vi "UHR-Fleezers Control (host) - 10.4.vi"() -> ()   [LabVIEW 2011] (continued)
  out "Progress":u16(slide) scale=0.0..100.0
  out "Manipulating Trap":bool
  out "Buffer Status":dbl(slide) scale=0.0..1.0
  out "Overflow (data lost)":bool
  in  "Reset":bool
  out "Data Rate (Hz)":dbl=66666.66666666667 caption="Trap Data Rate (Hz)" format="%#_3p"
  out "Data Period (s)":dbl=1.4999999999999999e-05 caption="Trap Data Period (s)" format="%#_6p"
  out "Save Data Rate (Hz)":dbl=133.33333333333334 caption="Rate (Hz)" format="%#_6p"
  out "Save Data Period (s)":dbl=0.0075 caption="Period (s)" format="%#_6p"
  in  "T1 alpha_x (nm/V)":dbl=624.3667930897869 step=10.0 format="%#_3g"
  in  "T2 alpha_x (nm/V)":dbl=812.659816494575 step=10.0 format="%#_3g"
  in  "T2 kappa_x (pN/nm)":dbl=0.20437519788264086 min=0.0 step=0.001 format="%#_2g"
  in  "T2 offset_x (mV)":dbl=53.075312649641084 format="%#_2g"
  in  "BD 1 Frequency 1 (MHz)":dbl=70.0 caption="T1 X (MHz)" min=60.0 max=90.0 step=1.0 format="%#_6p"
  in  "BD 1 Frequency 2 (MHz)":dbl=85.0 caption="T2 X (MHz)" min=60.0 max=90.0 step=1.0 format="%#_6p"
  in  "Green Laser ON/Interlacing":bool
  in  "Round T2 X":bool caption="Round"
  in  "AO1":dbl(slide)=7.146906643879515 caption="Confocal Y (V)" min=0.0 max=10.0 step=0.01 scale=0.0..10.0 scale format="%_1f"
  in  "AO2":dbl(slide)=1.424915616321299 caption="Confocal X (V)" min=0.0 max=10.0 step=0.01 scale=0.0..10.0 scale format="%_1f"
  in  "Trap Raster Scan":bool
  out "Raster Scanning...":bool
  in  "Trap Delta (MHz)":dbl=15.0
  in  "Setpoints (V)":cluster{"Set 1":dbl, "Set 2":dbl}={"Set 1"=9.0, "Set 2"=9.0}
  in  "Green FB Setpoint (mV)":dbl=200.0
  in  "Fish for Tether":bool
  in  "Position Label 5":string="upper flow spot (UvrD)" caption="5"
  in  "Move to Position":bool
  in  "Position":dbl=1.0 min=1.0 max=10.0 step=1.0
  in  "Set Position":bool
  in  "Saved Stage Positions":dbl[][](array[numeric])=[[1.0, 0.0, 0.0, 0.0], [2.0, -0.38428, -2.10668, -0.02109], [3.0, 1.5, -0.5, 0.0], [4.0, -0.59033, -2.08842, -0.03013], [5.0, 1.5, -2.25, 0.0], [6.0, 0.0, 0.0, 0.0], [7.0, 0.0, 0.0, 0.0], [8.0, 0.0, 0.0, 0.0], [9.0, 0.0, 0.0, 0.0], [10.0, 0.0, 0.0, 0.0]]
  in  "Move to Position 5":bool
  in  "z nudge increment (um)":dbl=0.5
  in  "+z":bool
  in  "Position 1 Label":string="Lower capillary (DNA beads)" caption="1"
  in  "Set Position 1":bool
  in  "Set Position 2":bool
  in  "Set Position 3":bool
  in  "Set Position 4":bool
  in  "Move to Position 3":bool
  in  "Move to Position 4":bool
  in  "Move to Position 2":bool
  in  "Move to Position 1":bool
  in  "Position 2 Label":string="Upper capillary (ADig beads)" caption="2"
  in  "Position 3 Label":string="lower flow spot (ATP)" caption="3"
  in  "Position 4 Label":string="Dump beads" caption="4"
  in  "-z":bool
  in  "Set Position 5":bool
  out "Stage Control Serial Error":errorcluster={"status"=FALSE, "code"=1073676293, "source"="VISA Read in Set Stage Position.vi->UHR-Fleezers Control (host) - 10.4.vi"}
  in  "Clear Volume":bool caption="Clear Infused Volume"
  in  "Flow rate (uL/h)":dbl=100.0
  in  "Flush rate (uL/m)":dbl=100.0
  out "Pump 3 cont disp":string="Left: ADig beads"
  out "Pump 1 cont disp":string="Right: DNA beads "
  in  "Ch 1 Inject Rate (ul/h)":dbl=1600.0
  in  "Pump write delay (ms)":dbl=300.0
  in  "All Pump Parameters":T5={"Pump 1"={"Diameter (mm)"=4.61, "Units"=4.0, "Volume"=100.0, "Rate"=1600.0}, "Pump 2"={"Diameter (mm)"=4.61, "Units"=3.0, "Volume"=0.0, "Rate"=0.0}, "Pump 3"={"Diameter (mm)"=4.61, "Units"=4.0, "Volume"=100.0, "Rate"=800.0}}
  in  "Ch 1 Inject Volume (uL)":dbl=100.0
  in  "Pump pause delay (ms)":u32
  in  "Ch 3 Inject Volume (uL)":dbl=100.0
  in  "Ch 3 Inject Rate (ul/h)":dbl=800.0
  in  "Flush Center Ch Volume (uL)":dbl=15.0
  in  "Flush Center Ch Rate (ul/m)":dbl=100.0
  in  "Inject Pump 2":bool caption="Inject Pump 2\n(Flush Center)"
  in  "Total Volume\nFlushed (uL)":dbl
  in  "Flush Sample":bool
  in  "Volume (uL)":dbl=100.0
  in  "Tab Control 2":T6(tab)=enum."Feedback on Trap Position"
  out "Total Counts (ticks)":u32=600
  in  "Trap ON/OFF X or Y Amp?":bool=TRUE
  in  "Oscillate Set 1":bool
  in  "Trap 1 ON":bool=TRUE
  in  "Number Interlace Sets":u8=3 min=1 max=3
  in  "DIO count 3 (ticks)":u32=200
  in  "DIO count 2 (ticks)":u32=200
  in  "DIO count 1 (ticks)":u32=200
  in  "BD 2 Amplitude 3 (%)":dbl min=0.0 max=50.0 step=1.0
  in  "BD 2 Amplitude 2 (%)":dbl min=0.0 max=50.0 step=1.0
  in  "BD 2 Amplitude 1 (%)":dbl min=0.0 max=50.0 step=1.0
  in  "BD 1 Amplitude 3 (%)":dbl min=0.0 max=50.0 step=1.0
  in  "BD 1 Amplitude 2 (%)":dbl=35.0 min=0.0 max=50.0 step=1.0
  in  "BD 1 Amplitude 1 (%)":dbl=10.0 min=0.0 max=50.0 step=1.0
  in  "BD 2 Frequency 3 (MHz)":dbl=26.0 min=0.0 max=40.0 step=1.0 format="%#_6p"
  in  "BD 1 Frequency 3 (MHz)":dbl=70.0 min=60.0 max=90.0 step=1.0 format="%#_6p"
  in  "BD 2 Frequency 2 (MHz)":dbl=26.0 min=0.0 max=40.0 step=1.0 format="%#_6p"
  in  "BD 2 Frequency 1 (MHz)":dbl=26.0 min=0.0 max=40.0 step=1.0 format="%#_6p"
  in  "Not-Interlacing Set":enum32{"Set 1", "Set 2", "Set 3"}(radio)
  in  "Interlace":bool=TRUE
  in  "Trap 2 ON":bool
  in  "Trap 3 ON":bool
  in  "Scan axis 2":bool=TRUE
  in  "Osc. freq. (Hz)":dbl=0.25
  in  "Osc. amp. (MHz)":dbl=2.0
  out "Coords":T7
  in  "Manipulation Scaling":cluster{"Horizontal":dbl, "Vertical":dbl}={"Horizontal"=0.075, "Vertical"=0.01}
  in  "Freq or Amp switch first":bool=TRUE
  in  "Swap F1 and F2":bool
  in  "Freq switch delay":u16
  in  "Amp switch delay":u16=5
  in  "MCL Step Increment (V_int)":dbl=3.0
  out "Time to Finish All (min)":dbl=0.13986 format="%#_2p"
  in  "Scan Speed (nm/s)":dbl=100.0
  in  "Scan Range (nm)":dbl=420.0
  in  "Step Size (nm)":dbl=1.0
  in  "MCL/AOM Scale Tweak":dbl=1.0
  in  "MCL Step Position Ratio":dbl=0.5
  in  "Move MCL Also?":bool=TRUE
  out "Final sep (nm)":dbl=1440.000000000001
  out "Initial sep (nm)":dbl=1020.0
  out "Save index":dbl=12.0
  out "Final delta (MHz)":dbl=18.41463414634147
  out "Initial delta (MHz)":dbl=15.0
  out "Final freq. (MHz)":dbl=66.58536585365853
  out "Initial freq. (MHz)":dbl=70.0
  in  "Saved AOD Raster Scan Parameter Sets":T8(array[cluster])=[{"Scan Range AOD (nm) 2"=500.0, "Step Size AOD (nm) 2"=1.0, "Scan Speed AOD (nm/s) 2"=100.0, "Number of scans (AOD) 2"=1, "Label"="offset curve"}, {"Scan Range AOD (nm) 2"=420.0, "Step Size AOD (nm) 2"=1.0, "Scan Speed AOD (nm/s) 2"=100.0, "Number of scans (AOD) 2"=1, "Label"="hp raster check"}, {"Scan Range AOD (nm) 2"=6.8, "Step Size AOD (nm) 2"=0.34, "Scan Speed AOD (nm/s) 2"=0.34, "Number of scans (AOD) 2"=1, "Label"="3.4 kbp - 1 bp steps"}, {"Scan Range AOD (nm) 2"=215.0, "Step Size AOD (nm) 2"=1.0, "Scan Speed AOD (nm/s) 2"=100.0, "Number of scans (AOD) 2"=3, "Label"="dt14 1 14 MHz start"}, {"Scan Range AOD (nm) 2"=450.0, "Step Size AOD (nm) 2"=1.0, "Scan Speed AOD (nm/s) 2"=100.0, "Number of scans (AOD) 2"=1, "Label"="dt14 2 small beads"}]
  in  "Load parameters":bool
  out "Scan Range (MHz)":dbl=-3.4146341463414633
  in  "Restart DMA? (AOD)":bool=TRUE caption="Restart DMA?"
  out "Incr. int (AOD)":i64=-7759651845
  out "Time/Scan (s) (AOD)":dbl=4.1958 format="%#_2p"
  out "Data points/scans":dbl=559440.0
  out "Data points/scan (f/b)":dbl=559440.0
  in  "Save scans":bool=TRUE
  out "AOD Scan I":u64=2 caption="Scan I"
  in  "Continuous AOD Scanning":bool caption="Continuous Scanning"
  in  "Abort AOD Scan":bool caption="Abort Scan"
  in  "Scan BD":bool=TRUE
  out "Cycles/step (AOD)":u64=666 format="%.3p"
  in  "Number of F/B Scans (AOD)":u16=1 min=1
  out "Scan steps (AOD)":u64=420
  out "Scan Increment (MHz)":dbl=-0.008149484836137144
  out "AOD Scanning":bool caption="Scanning"
  in  "Start AOD Scan":bool caption="Start Scan"
  out "N sets should be saved":dbl=27.972
  out "Progress 2":u16(slide) caption="Progress" scale=0.0..100.0
  in  "Abort save 2":bool caption="Abort save"
  in  "Trap 1 Bead Size (nm)":dbl=860.0
  in  "Trap 2 Bead Size (nm)":dbl=790.0
  out "MCL Count":dbl=782931.6080202643
  in  "All FB On/Off":bool=TRUE
  in  "AI2 to Setpoint":cluster{"Set 1":bool, "Set 2":bool}
  out "AI2 (V)":cluster{"Set 1":dbl, "Set 2":dbl}={"Set 1"=9.049958800012208, "Set 2"=0.022888882106997896}
  in  "Reset Feedback":cluster{"Set 1":bool, "Set 2":bool}
  in  "PID Gains":T9={"Set 1"={"proportional gain (Kc)"=0, "integral gain (Kc*Ts/Ti)"=5, "derivative gain (Kc*Td/Ts)"=0}, "Set 2"={"proportional gain (Kc)"=0, "integral gain (Kc*Ts/Ti)"=5, "derivative gain (Kc*Td/Ts)"=0}}
  in  "Feedback On/Off":cluster{"Set 1":bool, "Set 2":bool}={"Set 1"=TRUE, "Set 2"=TRUE}
  in  "Rem fb disp offset":bool caption="Rem. Offset"
  in  "Remove Unwinding Offset":bool
  in  "FB Trap Pos Offset":dbl=-32.20986371566535 caption="Offset (nm)" format="%.1f"
  in  "Negate Y Axis":bool=TRUE
  in  "Set Reading to\nSetpoint":bool
  out "Trap X (AI1)":T10={"Trap 1"=0.05029296875, "Trap 2"=-0.09722900390625}
  in  "Trap Pos FB SP":fxp<+/-,16,1>=-0.008514404296875 caption="Setpoint"
  in  "Trap Pos. FB ON":bool
  in  "Reset Trap Pos. FB":bool
  out "Trap Positions":waveform(dbl)[](graph)=[{"t0"=timestamp(5315.100000001762 s since 1904-01-01), "dt"=0.15, "Y"=[-32.20986371563738, -32.20986371563738], "attributes"=variant("NI_ChannelName"=variant(string "Trap 1 Pos."))}, {"t0"=timestamp(5315.100000001762 s since 1904-01-01), "dt"=0.15, "Y"=[-5.5933924159035087e-11, -5.5933924159035087e-11], "attributes"=variant("NI_ChannelName"=variant(string "Trap 2 Pos."))}]
  in  "Tab Control 8":enum32{"Main Setting", "Details"}(tab)
  in  "Trap Pos FB Int Count":u16=100
  in  "Trap Pos. FB Gains":T11={"proportional gain (Kc)"=10.0, "integral gain (Kc*Ts/Ti)"=10.0, "derivative gain (Kc*Td/Ts)"=0.0} {"proportional gain (Kc)" format="%.11g"; "integral gain (Kc*Ts/Ti)" format="%.11g"; "derivative gain (Kc*Td/Ts)" format="%.11g"}
  in  "Trap Pos. FB Offset Factor":i64
  in  "Trap Pos FB Negate Action":bool
  in  "Trap Pos. FB Mult Factor":i64=33554432
  in  "Trap Pos. AI1 X Pre-scale":u16
  in  "Trap Pos. FB Range":T12={"output high"=0.999969482421875, "output low"=-1.0}
  out "Trap Pos FB Int Signal":fxp<+/-,24,9>=-1.02886962890625 format="%.18g"
  out "Trap Pos FB Int-Norm Signal":fxp<+/-,16,1>=-0.010284423828125 format="%.16g"
  in  "Set SP Using...":bool
  in  "Trap Pos FB Monitor\nT1 or T2":bool
  out "Trap X AI1 (DMA)":T13={"Set 1"=0.05328369140625, "Set 2"=-0.139556884765625}
  in  "N El. to Ave.":dbl=10000.0
  out "Trap Pos FB Action":i64=23570
  out "Action (%)":dbl(knob)=71.93212683492538 scale=-100.0..100.0
  in  "Trap Pos. FB Out Scale 2^n":u8=25 caption="Action Scale Factor"
  out "Mean T1 Position (nm)":dbl=-32.20986371563738 caption="Mean T1 (nm)" format="%0.2f"
  out "Trap 1 Position RMS (A)":dbl caption="RMS (Ang)"
  in  "Remove Action Offset":bool
  in  "factor":dbl=0.8
  in  "Trap Pos. Disp. Downsample":dbl=10000.0 caption="Trap Downsample"
  in  "Tab Control 3":enum32{"Timing", "MCL Scan", "Analog Out"}(tab)
  out "APD 2 Gate Late Counter":u32
  out "APD 2 Gate Relative Phase":i16
  in  "Phase Adj. (APD 2 Gate)":i16=20
  in  "Initial Phase Adjustment (APD 2 Gate)":i16=55
  out "APD 1 Gate Late Counter":u32
  in  "- phase (APD 1 Gate)":bool
  in  "+ phase (APD 1 Gate)":bool
  out "APD 1 Gate Relative Phase":i16
  in  "Phase Adj. (APD 1 Gate)":i16=20
  in  "Initial Phase Adjustment (APD 1 Gate)":i16=60
  in  "Save APD Data\nwith Trap Data":bool=TRUE
  out "APD FIFO Elements Remaining":u32
  in  "- phase (APD Acq)":bool
  in  "+ phase (APD Acq)":bool
  out "APD Acq Late Counter":u32
  out "APD Acq Relative Phase":i16
  in  "Phase Adj. (APD Acq)":i16=20
  in  "Initial Phase Adjustment (APD Acq)":i16
  in  "Invert APD Gate":bool caption="Invert Gate"
  in  "APD Gate OFF Count":u32=450 caption="Gate OFF Count"
  in  "APD Gate ON Count":u32=150 caption="Gate ON Count"
  in  "APD Gate":enum32{"ON", "OFF", "Interlace"}(radio)=enum."Interlace"
  in  "APD Integration Time (s)":dbl=0.01 caption="Integration Time (s)"
  out "APD Acq Rate (Hz)":dbl=100.0 caption="Rate (Hz)"
  out "APD Samples/FIFO Acq.":dbl=30.0
  out "APD Elements/DMA read":u32=60
  out "APD Int. Count":u32=400000 format="%.0p"
  in  "+ phase (APD 2 Gate)":bool
  in  "- phase (APD 2 Gate)":bool
  in  "Tab Control 5":enum32{"PSD X", "PSD Y", "Other Data Channel"}(tab)
  out "Data map":dbl[][](graph)=[[0.001974800723796629, -0.0013307077949780925, 3.5478396375182556e-05, -0.0008656630334600533, 0.003722726291225046, 0.0009559614811579494, 0.0004067776954783719, -0.0005330988948040376, -0.001176093052158523, 0.0004508069091133665, -0.0009073488729753098, -0.0007052486419013018, 0.00020789655803253064, 0.0001241869508331131, 0.0037172511150124366, -0.0002939967002449287, -0.00015207858051379504, -9.320397918003548e-05, -4.818930038232472e-05, 0.0003043649821186849], [-0.001031665574705379, -0.0005831254477400646, 0.0012531205354473264, 0.0006867260941382034, 0.00039068341874680536, -0.0008665544113564399, 1.1155677774738132e-05, -0.0004058382977629158, -0.0007996984738111764, 0.0006720220745334646, -5.2295719559871024e-05, 0.0020160741300127927, 0.0011086934717958095, 0.00022784846412103992, 0.0014286413450522995, -0.000625478515904662, -0.00032260854393552883, 0.0014821578105266167, -0.0006624520387635512, -0.0008196499516340234], [0.0008707462370312414, 0.0008734847802455585, -0.0009375270569827855, -0.0005301325848379493, 0.0008581834048839196, -0.00038982434612128277, 0.003239773338572745, -0.00020397792231700303, 0.0007502371285024098, 0.0002674083017176036, 0.0006760027114216932, -0.0005268526629850034, -0.0008874403582654871, 0.0021340380967751838, 0.00038914081701392413, -0.000607773836931023, 0.00040958612136905335, -8.912906425596873e-05, -0.000978322721709446, -0.0004259412094274336], [0.0010167653949750284, -0.001227712955400397, -0.0005828111751727386, -0.00034681313733748873, 0.0011154140304214628, 0.0009698055107082625, 0.0003047086624579304, -0.000896404784165975, 0.0010714187743685885, 0.0003983374192823886, -4.912248607555678e-05, -1.2318516008092849e-05, 9.095897165929441e-05, 0.0015280892564470835, 0.0015086948659084063, -0.0002666063281217702, -0.00023529227277871242, -0.00036125092589777287, -0.0014159788458990696, -2.710729292442805e-05], [-8.167246872768262e-05, 0.0009598305190754163, 0.0003747131180220494, 0.0012690684222979877, -0.00034832954634158697, 5.649447215263457e-05, 0.0004890411957727576, -0.0007578336539554914, -0.00040934283442915705, 0.0007452279948579076, 0.00015620465662804465, 0.0018487220354370564, 0.0014080398272018054, -0.00041784730224639767, -0.0003903906172355312, -0.0003199149811349592, 0.00035618530065829087, -0.0006799972758753446, -0.0003889301678648796, -0.0005956701562327435], [0.0018039939622592623, 0.0005245361826948688, -0.0005290632683555431, 0.0013464225880901197, 0.0023697527260712757, 0.0011020235591090992, 0.00020697879433716562, 0.0018739219447031124, 0.002825452929761835, 0.0030107134581543785, 0.001314432526129752, 0.003128098021455577, 0.0014332438566350687, 0.001086276942514396, 0.001205303903834992, -0.00016582908036511657, 0.00012758730652683684, -0.0003758331663356629, 0.0005886822950795234, 0.0015518682379053797], [-0.00012651639952852573, 0.00021197244368694504, 0.0012350748934195559, 0.0018402525422088435, 0.002745478751245486, 0.004131110694033679, 0.002058549584611999, 0.0030582421647530425, 0.0065060720254878, 0.006794612607701507, 0.006405329109429012, 0.003716164207065463, 0.005962917409522268, 0.004495605148869885, 0.002525312567946067, 0.003950367441137721, 0.0005331096487246145, 0.0005060946339809289, 0.0014243473110138849, 0.001130596778785661], [0.00014317515011674618, -4.3424295646923145e-05, 0.0021662489428812357, 0.0016275554184984802, 0.0044439595354786605, 0.006738407040550086, 0.008417220923640046, 0.009134415922172245, 0.010893231488705402, 0.010754864224228526, 0.009867759374005268, 0.00977448539430105, 0.011384712936667093, 0.007850181445882674, 0.0049035327963239325, 0.002096154924260298, 0.0018045353737507733, 0.0029106523159805543, 0.0015888039103951976, -0.00029337209432822917], [-6.242457633829093e-05, 0.0020003421357321716, 0.0028905748718623366, 0.005805262190070683, 0.005457239966035112, 0.008151652936542866, 0.010661769245138245, 0.010013034688360692, 0.011681959513417765, 0.011787651652910437, 0.012849701365447398, 0.013247108197576025, 0.009902952347460825, 0.010133150788845132, 0.00519303847640039, 0.007478338034713532, 0.0031833479798268937, 0.0022832956688604434, 0.001597751335202657, -0.00045194294226618315], [0.0023892743065292922, 0.002788418472585368, 0.0014096575829616606, 0.0028285307437255253, 0.006547664768557391, 0.008189527623975616, 0.009923409965297099, 0.008729730333927745, 0.010911115966886872, 0.007250206225461674, 0.012011244746535098, 0.012114648129158977, 0.006188134462039724, 0.008630661024945556, 0.0048325127371069065, 0.004455811813470026, 0.0035707708675729033, 0.001610709369645243, 0.0011937522039525432, -0.0002811898121190214], [0.0013313724301020982, 0.004207468392898867, 0.0004238823129005421, 0.002540290831678132, 0.004835232640166063, 0.004649156180713865, 0.006515897058840856, 0.006071012094608348, 0.0046033051355698126, 0.0047374830880438975, 0.004401277240177894, 0.0055173176057941396, 0.00498442300252165, 0.005995404058491503, 0.004329924063900099, 0.001165380052032569, 0.0015694819993301344, 0.001370962547386529, -0.000718356874026457, 0.0004930969885946206], [0.0007383004922265653, 0.0016834709429263915, -0.0008928849142594358, 0.0013755982583879241, 0.0014542399912162388, -0.00025075833091892314, -7.932373244942046e-05, 0.001271525984554565, -0.0007015281269428645, -0.0002781348202945594, 0.0004305619557892593, -0.000393268977090386, -0.0013807321525476448, -0.0011120854522711778, -0.0012526443531265463, -0.0007103799938683556, 0.00026359582093472193, 0.0005478450898007638, 0.0007966009161969348, 0.0008488605880798546], [-0.0006949432143705978, -0.00016588866665113446, -0.001218132512769711, -0.0016486995032421162, -0.002052352437058867, -0.0030955094973178143, -0.0034356999971391824, -0.004112235032535816, -0.00451349506697353, -0.004312730844741325, -0.004585222836713357, -0.0036276805983766402, -0.0056953242102699185, -0.005274266429337645, -0.004033396006691108, -0.00340958527530643, -0.002796881124356951, -0.0016801545682360738, -0.0009622748561198863, -0.0011867292270050338], [-0.0005436808600952939, -0.0019479440314470386, -0.0026903437012143626, -0.0034403505050561124, -0.004033038493854955, -0.005225041591182969, -0.006195203353611577, -0.007221398787988425, -0.007674397521616515, -0.007826743194638278, -0.007851843691143582, -0.008151412410915878, -0.008438971204370885, -0.00694589908177172, -0.0059676262489851, -0.004340938642355187, -0.0031099452652213226, -0.0022546373251876592, -0.0010308829443490927, -0.0014974708117689896], [-0.0009274189424054265, -0.002138127375731672, -0.0026737111318357737, -0.0030086293103776004, -0.004755351904761902, -0.0063717866899584575, -0.007557662173002423, -0.00895879321670302, -0.009851076668324032, -0.00952797317375972, -0.00978920542842815, -0.009171197174548833, -0.009091846511606355, -0.0074285536789867775, -0.005715795285311283, -0.0037509920803341186, -0.0028624093112670744, -0.0022129920941549312, -0.0009720791869701506, -0.00016390418315424392], [-0.0015018318064477822, -0.0017596917287992495, -0.00207741061968108, -0.0026903744641973096, -0.0041201947077022065, -0.005274996223771535, -0.006513040069634409, -0.007783971720920169, -0.008530656465900947, -0.008719784166919617, -0.008256349729222363, -0.007911526634713803, -0.007165468186465685, -0.005980774285518301, -0.0018316320640932233, -0.002948253454365279, -0.0016667417434297858, -0.001528162213141902, -0.0005241575459133675, -0.0012236858424283167], [-0.0012499405267868005, -0.0014949456064733933, -0.0005767994494934392, -0.0019390056710758418, -0.0018245806637560231, -0.0023548230765676813, -0.003388576213734222, -0.005069998536190779, -0.005265703621062351, -0.005084448084065333, -0.004105054126884424, -0.004753543346726036, -0.003731520608271496, -0.0034133289571792536, -0.0017511601237870304, 0.0008871056640322357, -0.0011529307336766393, -0.0013407099980656642, 0.0009377924224138966, 0.00031192289272911525], [-0.0007659382756858993, -0.0013973355617842775, -0.0014877986835744633, 0.00041749867945347203, -0.0017879497288791138, -0.0017461211016140095, -0.00042106281643194336, -0.00240042527641399, -0.0027715352406898924, -0.002989958342722546, -0.0012324408099390687, -0.0024854611194643937, -0.0011302657470884901, -0.0017945254556017676, -0.001166777371192933, -0.00020259785412322874, -0.00035365864453670013, -0.0014081948228195636, 0.00011400500739779627, -0.0009539563152650239], [-0.0012878630018548405, -0.0010820599773619431, -0.0015337169051551813, -0.0015146294723753866, -0.0006589923538424275, -0.0016750992481219854, -0.001576087969159457, 0.0004328244822703884, -0.0022786776408459295, -0.002133994122819535, -0.0015778307998133155, -0.0014028718511365518, -0.0013807424864769138, -0.0008191475054933096, 3.5168875292561656e-05, 0.0009571839669838163, -0.000691413272029182, -0.0011611206136471761, -0.0009895515508372736, 7.57233001477349e-05], [-0.0010536742474643562, -0.000991182845883618, -8.324594723825736e-05, -0.0011865682873398067, -0.0009013329230006353, -0.00031821111543612273, -0.0009340415228278681, -0.0011215542488407536, -0.0016373711880167123, -0.0017927984163725607, -0.0007465993865808737, -0.0003217900827132992, -0.0003106344844355273, -0.0006176526466302833, -0.0008629016203903469, -0.00039522843832119365, 3.810751656546153e-05, -0.0011098721179525716, -0.0010990998825502283, 0.0008060003289936492], [-0.0011214348504638779, -0.0004237929177585575, -0.00047027427710285517, -0.0007127568150182082, -0.001283624998445688, 0.000202027033119912, -0.00010337127679753888, -0.0006784694673924103, -0.0010469642464066464, -0.0005745771964042468, -0.0013717029285019958, -0.0003581026444660475, 0.0007592138461508972, -0.0008523248781440482, 0.0002286000011018851, -0.0007841396029935831, -0.00044419891417113596, 0.0003109908903585586, -0.0010818275324759156, -0.001051356913606505], [0.0004785726626459733, 0.0005220391204801982, -0.0005463478483528428, -0.0010449992873283482, -0.0007483617087881684, -0.001027059545965463, -0.0017679703661406486, -0.0015700380539653172, -0.0010506773864503213, 0.00029968871242246216, -0.0012099448373231428, 0.0001368549206433757, -0.0007538824633460659, -0.0007610585726775183, 0.0003755350646206948, 0.0009116135397215209, 0.0006653432025751911, -0.0009271047385618553, -0.00070345500978979, -0.00041502630335628045], [-0.0007263272368303678, -0.0003748943208977825, -0.0008472068029787485, -0.0010921258041779098, -0.0010655051920611374, -0.0010282217644289092, -0.0013000152541475425, -0.000961866962882997, 0.00011187603311087473, -0.0008839679006672069, -0.00046066837515954244, 0.0007782318940983726, -0.0004701832068316709, 0.001693289664051489, -0.0003305305837321905, 5.227664980688205e-05, 0.0007521242607856794, 0.00012791099420669656, -0.0009634753670072725, -0.0001804186018632445], [0.0016404591673853607, -0.0006620229264530011, -0.0007854812002567829, -0.0003104613980677611, -0.0005048032361081665, -0.000806896152924977, -0.000296311694344037, -0.00022878812776351822, 0.0009325154327282748, 0.001988875409334235, 0.0012075682350083787, 0.002925019733949366, 0.00047775383598309994, 0.0015812303905823678, 0.0006537826866560828, 0.0010221543400510279, 0.000538271490048766, -0.0003740502462371051, -0.00018291178926432023, 0.0003443347057549758], [0.002093818251619911, -0.0008952984395350009, -0.0004372574007258646, -0.0002286644695979288, 0.0008982068040037238, 0.0006097955197538334, 0.0007564768164306582, 0.0015231382339332723, 0.0018846718953476624, 0.0035285507222391696, 0.0033767791950066097, 0.002943241502325224, 0.003464381882164839, 0.0020346598064557783, 0.002543110601092136, 0.0012044713534041227, 0.0006147001856902608, 9.838811204051824e-05, -0.0004711361705212557, 0.0005440468312404789], [-0.0007122933932404857, 0.0006549111564878095, 0.00012015356188401353, 0.0011339179161487453, 0.0012605115663881024, 0.001846566333340279, 0.0027050543902905765, 0.0036763031317191075, 0.0038668575826173233, 0.004551503128127669, 0.004776421357772621, 0.004468868330278527, 0.004401441526203816, 0.004056102379065066, 0.0029356741196946306, 0.0024522350296070266, 0.0015803078332468634, 0.00110892109871749, 4.4364093684082584e-05, -0.0003486026777604606], [0.0008763494286269637, 0.0018712950591817997, 0.0006505291651649153, 0.0016703685555822228, 0.0031612238113091413, 0.0026322262228780143, 0.003508425855448398, 0.003833827324507288, 0.004168914019112371, 0.004236391265409293, 0.004612477759503962, 0.004464772410345458, 0.004153136308652595, 0.004183463770097493, 0.0036662929202140745, 0.002949190918155526, 0.002187722044198632, 0.0010302544922438455, 0.0003654092780044707, 0.0005862102844657458], [-1.3267658388671564e-05, -0.0001579958936313711, 0.0018705934115580756, 0.0015182354360879235, 0.001733212732566589, 0.002035957990177165, 0.0028035117877418304, 0.002360258553543087, 0.0026989294651921787, 0.0028199461162077763, 0.002859854487034166, 0.0025486274932714817, 0.0025574093637128776, 0.002857261171638578, 0.004003768191873129, 0.002769631468313185, 0.0023735237571786616, 0.0010887378578438847, -1.0076168635008711e-05, 0.0015870951719137506], [7.252799125267859e-05, -0.0004367990506991141, 0.0011465433397477947, 0.002640441619358938, 0.0009788721379060783, 0.0013080309928762478, 0.0015677671123940414, 0.0010695064182156691, 0.00240686193491007, 0.0036561067193890792, 0.0011200143541246275, 0.0018119022016169109, 0.0011010802122444654, 0.001678191345578103, 0.0013254823250920776, 0.001489379896239562, 0.0009861928951096725, 0.003166083569879477, 0.00034598282288794485, 0.00011835905027119764], [-0.0008744378810498419, -0.0006874739858229466, -4.684951587119415e-05, -0.00014428030246354617, -0.00019666010201344465, -0.00012021831250326627, 0.0006227708354450297, -0.00024135231533288466, 0.002043299595951369, 0.001206197500995257, -6.793762802426811e-05, 0.003309856561393797, 0.0009818104965593029, -0.0002214659499187642, 0.001441263674786213, -8.294342979673792e-05, 0.00012723757799097376, -0.00011734458359061474, -0.0008536473811964248, -0.0005289882386110797], [-0.0008927164030671517, -0.0003670390368122644, 0.0015231932352578214, -0.0005919163509102057, -0.0010622247823444493, -0.0004254284443583992, -0.0011519341993085786, -0.0003369266603182134, 0.0012453186232965125, -0.0017412013063361007, -0.0015608308766618688, -0.001471830504109942, -0.0021621309678003997, -0.0016219947676663943, 0.0004934040488059158, -0.000730820901741994, 0.0002799853416732386, 0.0008689916142481776, 0.0006503771397616425, -0.0006473720307864811], [-0.0010355722619993985, -0.00012330709791922418, -0.0011254876468762727, 6.374882001265107e-05, -0.0018420937214236345, -0.0015578797156731877, -0.0024958145067506066, -0.0018895680619412875, 0.00045034938468826004, 0.0001724258320007633, -0.0019512284899031742, -0.0013082623536610487, -0.0005665210030670095, -0.000402933592147318, 0.0006656573883463756, -0.002634710316370357, -0.0007595589979984393, 0.0003577529562837517, 0.0009785798074254841, -0.0009184376690793683], [0.00013439155652726403, -0.001569906431160574, -0.0016578235545035174, -0.0008488376175397862, -0.0027903469575648824, -0.001845541960481978, -0.00031682440085302834, -0.004341284339014073, 0.0009667888118025644, -0.001511940551895914, -0.0007208508194228646, -0.004318362814688104, -0.003488079823980268, -8.200742924438596e-05, -0.0006409042856662655, -0.0014662496530380446, -0.0025614437614861502, -0.0002966260235245425, 0.0012520699416297663, -0.0012102415905063644], [0.00018138614837264817, -0.0006319186284002348, 0.0005870634806117122, -0.001045825555779319, -0.0030834598381178522, -0.0006354170080386228, -0.0007868765145618403, -0.0030988815518741965, -0.0025865088152402646, -0.00106799061332729, -0.0018277279809409204, -0.0022237595271429374, -0.000914929178315798, -0.00195910452587799, -0.004054180535908664, -0.0016574896528336127, 0.00022115949014610986, 0.00023200317718135059, 0.0004442190952981046, -0.0008942827173167255], [-0.001376507083756199, -0.00029975861740799486, 4.049398152731954e-05, -0.0018876560919591162, -0.0008365269984459395, -0.00022319669640759082, -0.0021169358350621474, -0.0025756468784094598, -0.001456519331876108, -0.0025526993136919794, -0.001865550950241, 0.0009334517102777955, -0.003304644659532123, -0.001069667392341748, -0.002936280974240923, -0.001380981903818669, 0.0005029733727736563, -0.0007692010521565124, -0.0014773664751220725, 0.0006072658085879681], [-0.0013317540978594713, -0.001242907407943417, -0.0012482254898830716, -0.0014610500413196384, 0.0016649014090128447, -0.0012036857690772642, -0.0010561305200611469, -0.0005265355926507417, 0.0010216107642962377, -0.0031714982712575017, -0.001115399816003912, -0.0014075115025048712, -0.0018188062942410953, -0.000597466545218191, -0.0017117715888698276, 0.000847391326848181, 0.0005660659967269794, 0.0003681193242965745, 0.0011116300968026698, -6.130007866075708e-06], [-0.0013448394668393586, -0.0013216329317761325, -0.0005258569177200809, 0.00017181433993935418, -0.0006215087775820313, -0.0012440745025882791, -0.000775083624115995, -0.0019182454474208524, -0.0013105415517859595, -0.00022817927991505968, -0.0007936423338275054, -0.0011467203449001637, -0.0003041169163284585, -0.0012574691095254263, -0.0004081964292877671, -0.0011524413964498525, -0.0009737175716231466, -0.0010287589481518394, -0.0008314205726569729, -0.0007183215671026301], [0.0012189917717514587, -0.0015010657484751805, -0.0012099620699764614, 0.002315492481594202, -0.0008332627312661832, -0.0013077439765289526, -0.0015970501891621088, -0.0004940148180008931, 0.002630323242026012, -0.001121902293396304, -0.000212873895317427, -0.0010144090103719324, 9.979504428098359e-05, -0.0008545620539377942, 0.0015421122208716985, -0.000818249196775749, 0.00040062764884791645, -0.001010315097102947, -0.0009502370622879603, 3.2594299332581366e-05], [-4.119719831831303e-05, -0.0011402334759329606, -0.001846867209344832, 0.0003744330778655776, 0.00010425475265996629, -0.001742836885905614, -0.0016786889147864556, -0.0007980621600698947, -0.0010477063549030395, 7.576033015784959e-05, 0.001470698430638348, -0.0013827118690157355, 0.0009289999710756531, 0.000813951002037832, -0.0012974664732201746, -0.0005049085192115013, 0.0008556337126460953, 0.0018600031531098428, -0.001244393017199389, -0.0010590970127767989], [0.0005702808878649288, -0.0008791929966152144, 0.001132078143966701, 0.0013373662971268288, -0.0013223783182575123, -0.0010320905589294303, 0.001341054423952067, 0.0009145177427693996, 0.002348674640697923, -0.00016393274513426057, -0.0008172553050048459, -6.01602727050507e-05, 0.0013113335652848936, 0.0007537844812587035, -0.0010068052033608142, -0.0003562437521101122, -0.00039256227183823763, 0.0009728063715731054, -0.0011788717333510168, -0.0006925394556222149]]
  in  "Channel":i32=4
  in  "Abort MCL Scan":bool
  out "MCL Scan I":u64=21
  out "MCL Scanning":bool
  in  "Start MCL Scan":bool
  out "wait to reset values":bool
  in  "Tab Control 4":enum32{"Scan Settings", "MCL FPGA Loop Timing"}(tab)
  out "Total Time (s)":dbl=48.0
  in  "Scan lines (y)":u64=20
  in  "Fast Scan Dir":bool=TRUE
  in  "2D or 1D Scan":bool=TRUE
  out "Initial X":dbl=-0.2990749839777824
  out "Initial Y":dbl=6.251798760948517
  out "Time/f+b scan (s) (MCL)":dbl=2.4 caption="Time/scan (s)"
  in  "Number of scans (MCL)":u64=1 caption="Scans"
  in  "Scan steps (MCL)":u64=40 caption="Scan steps (x)"
  in  "N APD Samp/step":dbl=3.0
  in  "Scan Range (V)\n(of steps)":dbl=3.5
  in  "Restart DMA? (MCL)":bool=TRUE caption="Restart DMA?"
  in  "Continuous MCL Scanning":bool caption="Cont. Scanning"
  in  "Center Scan":bool=TRUE
  in  "Save Data (MCL)":bool=TRUE caption="Save Data"
  out "Actual Incr. int (MCL)":i16=294 caption="Incr. int"
  out "Desired incr (int)":dbl=294.0628205128205
  out "Desired Scan Incr (V)":dbl=0.08974358974358974
  out "N sets should be saved (MCL)":dbl=160.0 caption="N sets should be saved"
  out "Data points/scans (MCL)":dbl=4800.0 caption="Data points/scans"
  out "Data points/scan (f+b)":dbl=240.0 caption="points/scan (f+b)"
  out "Cycles/step (MCL)":u64=2000 caption="Cycles/step" format="%.0p"
  out "Actual MCL Inc (V)":dbl=0.08972441785943175
  in  "Phase adjust (MCL)":i16 caption="Phase adjust"
  out "Relative Phase (MCL)":i16 caption="Relative Phase"
  in  "Initial Phase Adj. (MCL)":i16 caption="Initial Phase Adj."
  in  "Update Count (MCL)":u32=600
  in  "+ phase (MCL)":bool
  in  "- phase (MCL)":bool
  out "MCL Late Counter":u32
  in  "APD 1 AO Mult.":i16=1 min=1
  in  "APD 2 AO Mult.":i16=1 min=1
  in  "Tab Control 7":enum32{"Green FB Signals", "Slow MCL Scan"}(tab)
  out "Green FB Plot":dbl(graph)=-0.012512588885158849
  out "MCL Scan 2":cluster{"Begin (V)":dbl, dbl, dbl[]}(graph)
  out "MCL Scan":cluster{"Begin (V)":dbl, dbl, dbl[]}(graph)
  in  "Green laser mode":enum32{"Laser ON", "Laser OFF", "Interlace"}(radio)=enum."Interlace"
  in  "GI Frequency, ON count":u32=150 min=1 step=1
  in  "Invert GI":bool
  out "GI Late Counter":u32
  in  "Phase adj. (GI)":i16=5
  out "GI relative phase":i16
  in  "+ phase (GI)":bool
  in  "Initial Phase Adjustment (GI)":i16=19
  in  "GI Frequency, OFF count":u32=450 min=1 step=1
  in  "- phase (GI)":bool
  out "Green FB Signals (V)":cluster{"Y":dbl, "X":dbl, "Sum":dbl}={"Y"=-799.1951219512196, "X"=-799.1951219512196, "Sum"=-0.012512588885158849}
  out "Relative phase (Green FB)":i16
  in  "+ phase (Green FB)":bool
  in  "- phase (Green FB)":bool
  out "Green FB Count":u32=600
  in  "Phase adj. (Green FB)":i16=10
  in  "Initial Phase Adjustment (Green FB)":i16=50
  in  "Green FB On/Off":bool=TRUE
  in  "Current When FB OFF (%)":dbl=87.0 min=0.0 max=100.0 step=1.0
  in  "Green int current ON count adj":u32=150
  in  "Green FB Gains":T14={"proportional gain (Kc)"=10, "integral gain (Kc*Ts/Ti)"=5, "derivative gain (Kc*Td/Ts)"=0}
  in  "- phase (GI) 2":bool
  in  "Initial Phase Adjustment (GI) 2":i16=-100
  in  "+ phase (GI) 2":bool
  out "GI relative phase 2":i16
  in  "Phase adj. (GI) 2":i16=20
  out "GI Late Counter 2":u32
  in  "On one out of X cycles":u32=1
  in  "Trap Position FIFO Depth":u32=300000 format="%.0p"
  in  "# Samples/trap":u32=20000 format="%.0p"
  out "Trap AI Elements/DMA read":u32=320000 format="%.0p"
  out "Ave. Rate (Hz)":dbl=200000.0 format="%#_6p"
  out "FIFO El. Rem.":u32 format="%.0p"
  in  "Phase adj. (AI1)":i16=15
  out "Relative phase (AI1)":i16
  in  "+ phase (AI1)":bool
  in  "- phase (AI1)":bool
  out "Late Counter (AI1)":u32
  in  "Initial Phase Adjustment (AI1)":i16=220
  out "AI rate (Hz)":dbl=200000.0 format="%#_6p"
  in  "AI Count (ticks)":u32=200
  out "# Samples/channel":u32=40000 format="%.0p"
  in  "Trap AI FIFO Depth":u32=600000 format="%.0p"
  in  "Detector Type":string(combo)="IR-QPD + PSD + FB-QPD X position"
  in  "N Acq Sets (Traps + Fl.)":i16=3
  in  "Sets to FIFO (Traps)":T15={"Set 1"=TRUE, "Set 2"=TRUE, "Set 3"=FALSE}
  in  "FPGA Ave.":dbl=1.0 min=1.0 step=1.0
  out "Ave. Period (s)":dbl=5e-06 format="%#_6p"
  out "DMA Update Period (s)":dbl=0.3
  out "FPGA Averaging":bool
  out "Trap Sets":u32=2
  out "Counts/DMA":dbl=12000000.0 format="%#_6p"
  out "Trap Pos FIFO El Remaining":u32=258
  out "Trap Pos Elements/DMA read":u32=120000 format="%.0p"
  out "Trap AI FIFO Timeout":u16
  out "Trap Pos FIFO Timeout":u16
  in  "Video Capture Rate (Hz)":dbl=30.0
  in  "Video Index":dbl=1.0 min=1.0 step=1.0
  in  "New Video File":bool
  in  "Save Video":bool
  in  "Reset Averaging":bool
  in  "Averaging":bool
  in  "Save Image":bool
  in  "Image Index":dbl=1.0 min=1.0
  out "Path Out":path
  in  "Center Point":cluster{"X":i32, "Y":i32}={"X"=335, "Y"=271}
  in  "Zoom Factor":sgl=7.0
  out "Window Size":cluster{"Width":i32, "Height":i32}
  out "Window Position":cluster{"X Position":i32, "Y Position":i32}={"X Position"=40, "Y Position"=40}
  in  "Initial Window Size":cluster{"Width":i32, "Height":i32}={"Width"=884, "Height"=619}
  in  "Initial Window Position":cluster{"X Position":i32, "Y Position":i32}={"X Position"=796, "Y Position"=4}
  in  "Intensity Upper":dbl=88.0
  in  "Intensity Lower":dbl=66.0
  out "error out":errorcluster
  out "error out 2":errorcluster
  in  "Harvard Syringe Pump Serial Port":refnum<visa-resource-name>="ASRL5::INSTR"
  in  "Lost Tether Alarm Threshold (pN)":dbl=0.5
  in  "AOM X Cal (nm/MHz)":dbl=123.0
  in  "MCL X Cal (nm/V)":dbl=1070.0
  out "X RF Amplitude Limits (%)":T16={"Minimum"=0.0, "Maximum"=50.0, "Increment"=1.0}
  out "X RF Frequency Limits (MHz)":T16={"Minimum"=60.0, "Maximum"=90.0, "Increment"=1.0}
  out "Y RF Frequency Limits (MHz)":T16={"Minimum"=0.0, "Maximum"=40.0, "Increment"=1.0}
  out "Y RF Amplitude Limits (%)":T16={"Minimum"=0.0, "Maximum"=50.0, "Increment"=1.0}
  in  "Manip. X?":bool=TRUE
  in  "Manip. Y?":bool
  in  "Force Manip Abort":bool
  out "Read cal error":errorcluster
  in  "DAQ Delay (ms)":u32=1000
  in  "Start Scan":bool
  in  "Scan axis":bool=TRUE
  in  "Osc. amp. (V)":dbl=5.0
  in  "Osc. center (V)":dbl=5.0
  in  "Osc. freq. (Hz) 2":dbl=1.0
  in  "MCL Mode":u16(ring) items=["Manual Positioning", "Sinusoidal Wave", "Linear Scan"]
  in  "Begin (V)":dbl
  in  "End (V)":dbl=10.0
  in  "N Points":dbl=20.0
  in  "Delay to Interlace (s)":dbl
  in  "Delayed Interlace Start":bool
  in  "Read Lateness and Rel Phase":bool
  out "Vec Mean of T1 T2":dbl[](array[numeric])=[15.284788421061677, 15.351412345296211]
  in  "Cal read wait (s)":u32=5
  out "Time tether formed":timestamp=timestamp(3395148454.934387 s since 1904-01-01)
  in  "Sample Chamber Stage Serial Port":refnum<visa-resource-name>="ASRL4::INSTR"
  in  "Chemyx Syringe Pump Serial Port":refnum<visa-resource-name>="ASRL3::INSTR"
  in  "Limit Min (MHz)":dbl=10.0 caption="Min (MHz)"
  in  "Limit Max (MHz)":dbl=16.0 caption="Max (MHz)"
  in  "Limits Enable":bool=TRUE caption="Enable"
  out "AI labels":string[](array[string])=["T1 Y", "T1 X", "T1 Sum", "T2 Y", "T2 X", "T2 Sum", "T1 FB X", "T1 FB Sum", "T2 FB X", "T2 FB Sum", "PSD Y", "PSD X", "PSD Y Sum"]
  in  "Save Trap Pos. Data":bool=TRUE
  # "After"
  # "During"
  # "Trap On?"
  # "BD Flow ON?"
  # "Samp Flow ON?"
  # "Trap Trig. Fl.?"
  # "Zero It"
  # "Floor it\n(e.g., hp unwinding)"
  # "1"
  # "2"
  # "Trap Display:"
  # "APD Display:"
  # "DAQ"
  # "Trap Manipulation"
  # "Data Saving"
  # "Bead Calibration"
  # "Chemyx Pumps\n(for bead syringes)"
  # "Harvard Pump\n(sample channel for flow exp)"
  # "Chemyx Pump 2"
  # "Units: \n1 = ml/m\n2 = ml/h\n3 = ul/m\n4 = ul/h"
  # "Rate param is ul/h\nVolume param is ul"
  # "X"
  # "Y"
  # "Oscillate Set 1 freq. (debugging)"
  # "BD 1"
  # "BD 2"
  # "AOD Raster Scan"
  # "Approx. trap separations"
  # "X"
  # "Y"
  # "FPGA\nreading"
  # "DMA\ntransfer"
  # "APD Gates"
  # "APD 2"
  # "APD 1"
  # "X"
  # "2D"
  # "Y"
  # "1D"
  # "Green Laser Interlacing"
  # "Green FB Measurement"
  # "Digital Gate"
  # "Current Analog Control"
  # "Total AI Rates (NOT rates/trap)"
  # "(Samples/trap x Trap Sets)"
  # "(Samples/channel x\n8 if averaging (8 channels)\n4 if no averaging)"
  # "Trap 1"
  # "Trap 2"
  # "Flour./Trap 3"
  # "External Video Window"
  # "MCL Position Debugging"
  # "Temporary Control Storage\n(these used to be somewhere else, still want to keep them)"
  # "Y"
  # "X"
  # "Trap Position Difference Limits"
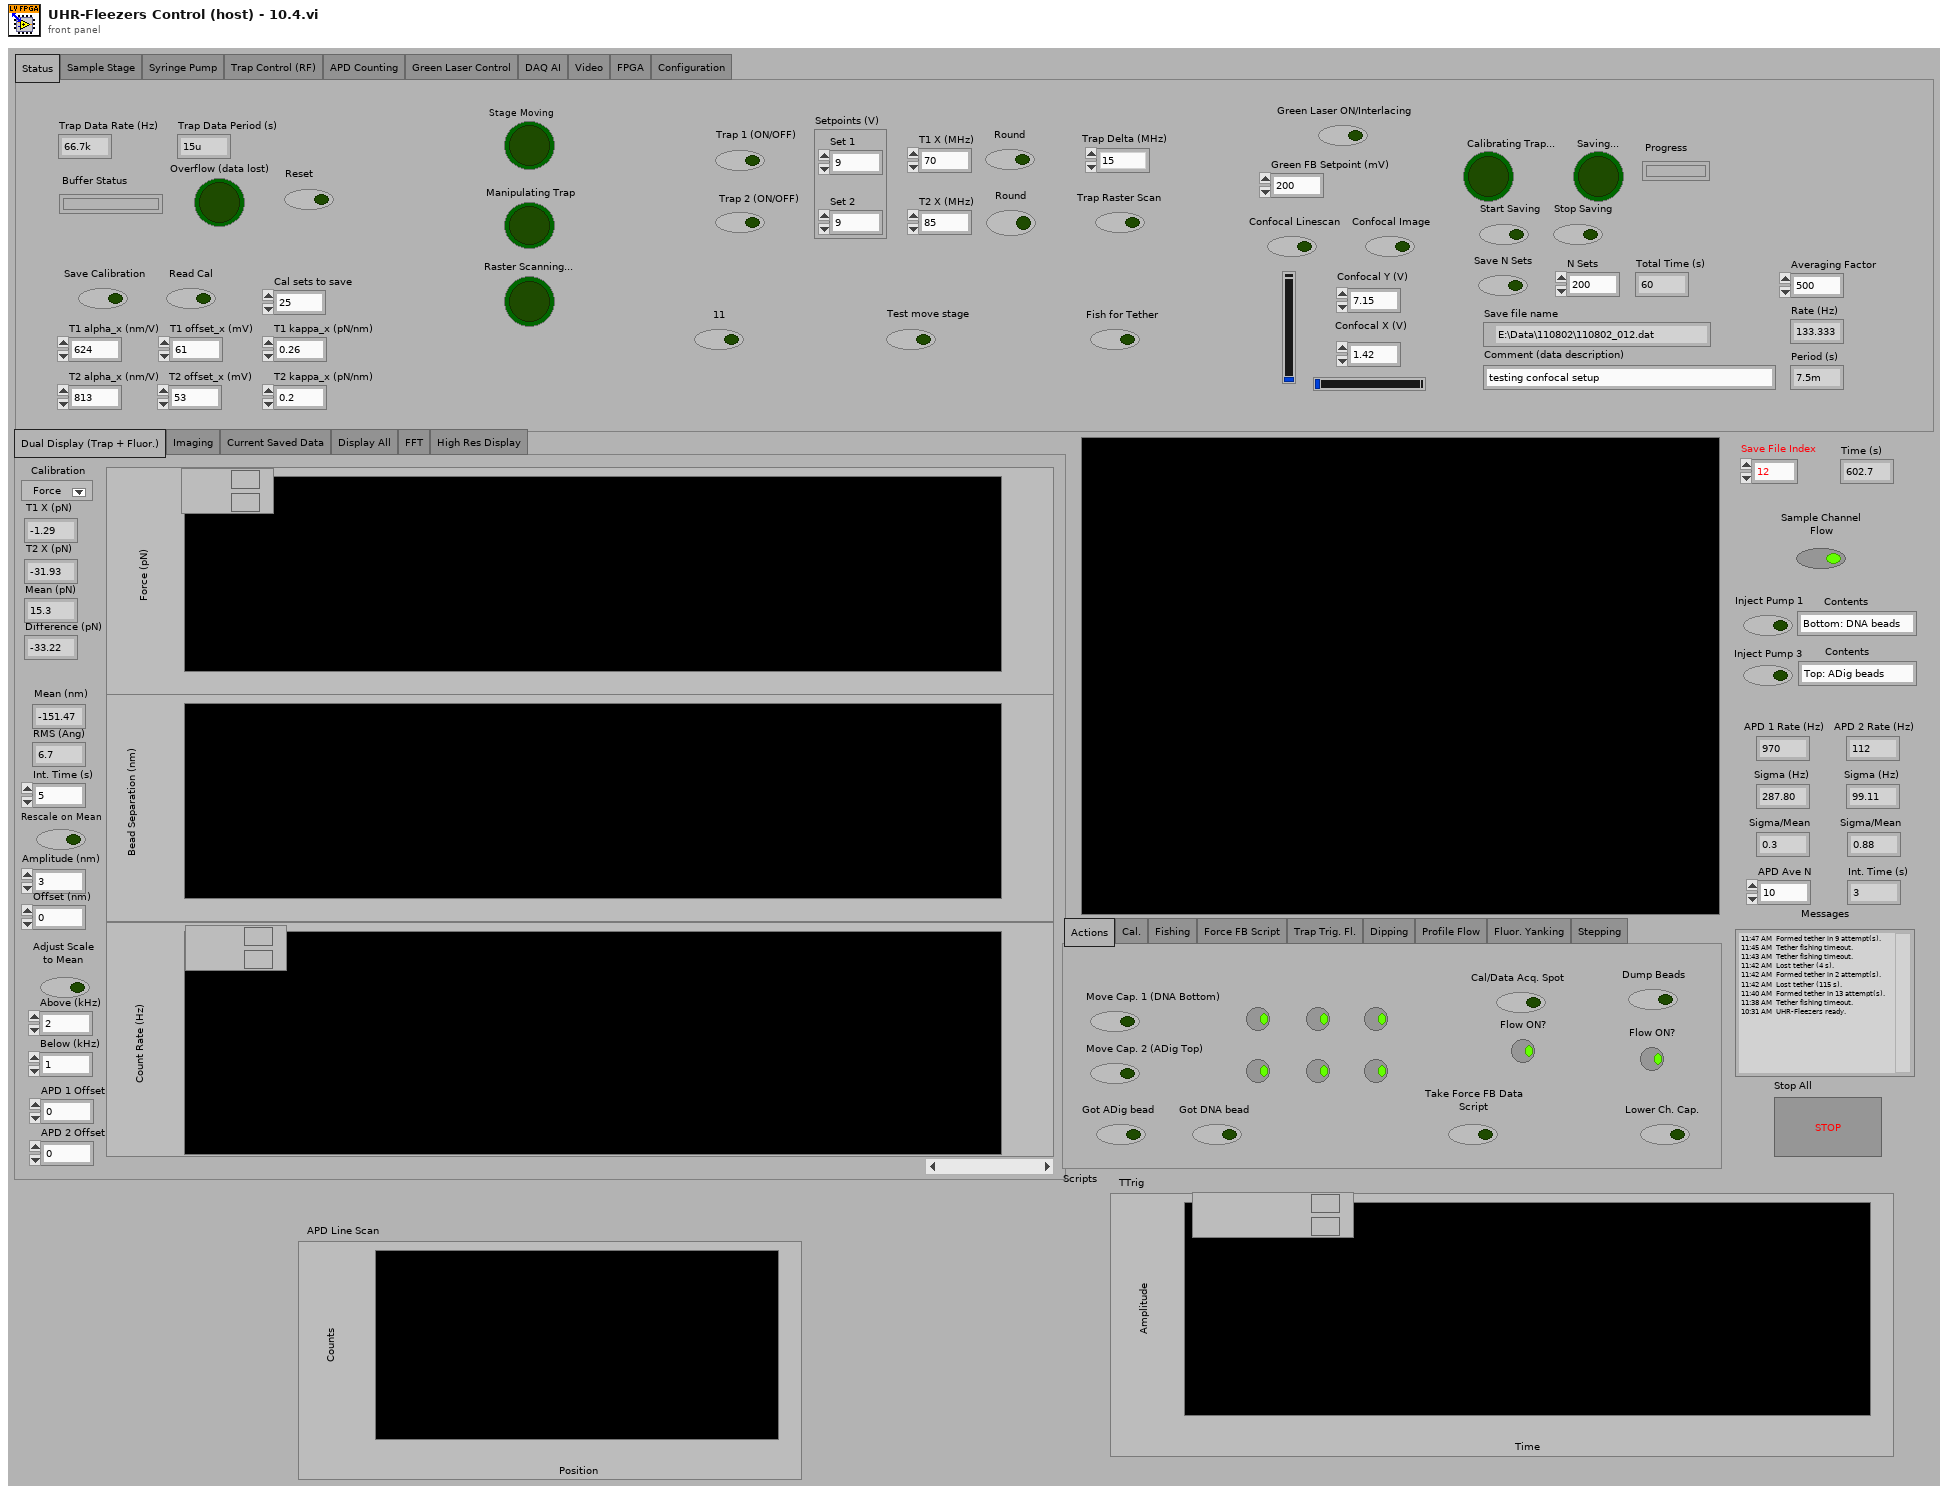
[diagram p1: front panel]
types:
  T1 = enum32{"Actions", "Cal.", "Fishing", "Force FB Script", "Trap Trig. Fl.", "Dipping", "Profile Flow", "Fluor. Yanking", "Stepping"}
  T2 = typedef "IMAQ Image.ctl" = refnum<image>
  T3 = enum32{"Dual Display (Trap + Fluor.)", "Imaging", "Current Saved Data", "Display All", "FFT", "High Res Display"}
  T4 = enum32{"Status", "Sample Stage", "Syringe Pump", "Trap Control (RF)", "APD Counting", "Green Laser Control", "DAQ AI", "Video", "FPGA", "Configuration"}
  T5 = cluster{"Pump 1":cluster{"Diameter (mm)":dbl, "Units":dbl, "Volume":dbl, "Rate":dbl}, "Pump 2":cluster{"Diameter (mm)":dbl, "Units":dbl, "Volume":dbl, "Rate":dbl}, "Pump 3":cluster{"Diameter (mm)":dbl, "Units":dbl, "Volume":dbl, "Rate":dbl}}
  T6 = enum32{"IR Laser Interlacing (Direct RF Board Control Method)", "AOD Raster Scan", "Feedback on Trap Intensity", "Feedback on Trap Position"}
  T7 = typedef "LVPoint32TypeDef.ctl" = cluster{"Horizontal":i32, "Vertical":i32}
  T8 = cluster{"Scan Range AOD (nm) 2":dbl, "Step Size AOD (nm) 2":dbl, "Scan Speed AOD (nm/s) 2":dbl, "Number of scans (AOD) 2":u16, "Label":string}[]
  T9 = cluster{"Set 1":cluster{"proportional gain (Kc)":i16, "integral gain (Kc*Ts/Ti)":i16, "derivative gain (Kc*Td/Ts)":i16}, "Set 2":cluster{"proportional gain (Kc)":i16, "integral gain (Kc*Ts/Ti)":i16, "derivative gain (Kc*Td/Ts)":i16}}
  T10 = cluster{"Trap 1":fxp<+/-,16,1>, "Trap 2":fxp<+/-,16,1>}
  T11 = cluster{"proportional gain (Kc)":fxp<+/-,16,8>, "integral gain (Kc*Ts/Ti)":fxp<+/-,16,8>, "derivative gain (Kc*Td/Ts)":fxp<+/-,16,8>}
